vi "SwapInstanceVIUnusedName2 69.vi"(6 "Bindata & descr in":T1, 7 "type":cdb, 8 "error in (no error)":errorcluster, 9 "dims":u8=3 min=1 max=3, 11 "kwarg_name":string="testarg") -> (0 "error out":errorcluster, 1 "Array 3D":cdb[][][](array[numeric]) format="%.2f", 2 "Array 2D":cdb[][](array[numeric]) format="%.2f", 3 "Array 1D":cdb[](array[numeric]) format="%.2f", 4 "Bindata & descr out":T1, 5 "bindata":u8[](array[numeric]))   [LabVIEW 2018]
uses:
  Bindata&description.ctl
  Bindata description.ctl
  bdcbfef1-0b46-4e56-956b-efd7e52a8352.vi
  ec4bf352-c22a-4021-8efd-577ac70aacaa.vi
  66b8b619-fbe3-45a4-a1cc-203eb9b1f5dc.vi
  f262bfa0-5f14-49db-af0c-aad155b06c38.vi
  ec4bf352-c22a-4021-8efd-577ac70aacaa.vi/961f97e1-d54a-4e62-be37-74572e5b9f83.vi
  66b8b619-fbe3-45a4-a1cc-203eb9b1f5dc.vi/5bdaa807-7911-40a4-928e-6d0b25e11cf6.vi
  f262bfa0-5f14-49db-af0c-aad155b06c38.vi/a331fc70-2e34-4be0-817e-a64d7f4c7d79.vi
  ec4bf352-c22a-4021-8efd-577ac70aacaa.vi/961f97e1-d54a-4e62-be37-74572e5b9f83.vi/a85859f1-6a01-45ef-8e4c-231faaeaae98.vi
  66b8b619-fbe3-45a4-a1cc-203eb9b1f5dc.vi/5bdaa807-7911-40a4-928e-6d0b25e11cf6.vi/e5bad492-59a7-411a-a4a3-726d696f4125.vi
  f262bfa0-5f14-49db-af0c-aad155b06c38.vi/a331fc70-2e34-4be0-817e-a64d7f4c7d79.vi/75280eb0-2824-4b96-8a24-41904d7d4e2c.vi
  ec4bf352-c22a-4021-8efd-577ac70aacaa.vi/961f97e1-d54a-4e62-be37-74572e5b9f83.vi/a85859f1-6a01-45ef-8e4c-231faaeaae98.vi/9d1e86aa-c211-4185-9eac-3e06c0eb4835.vi
  66b8b619-fbe3-45a4-a1cc-203eb9b1f5dc.vi/5bdaa807-7911-40a4-928e-6d0b25e11cf6.vi/e5bad492-59a7-411a-a4a3-726d696f4125.vi/91efaebe-290b-41fc-a773-0eb7a6083b7d.vi
  f262bfa0-5f14-49db-af0c-aad155b06c38.vi/a331fc70-2e34-4be0-817e-a64d7f4c7d79.vi/75280eb0-2824-4b96-8a24-41904d7d4e2c.vi/24bfebee-2e4b-4f78-9251-0a951621d460.vi
  check ID validity.vi
  LV-Julia_ZMQ-Roundtrip_lib.lvlib
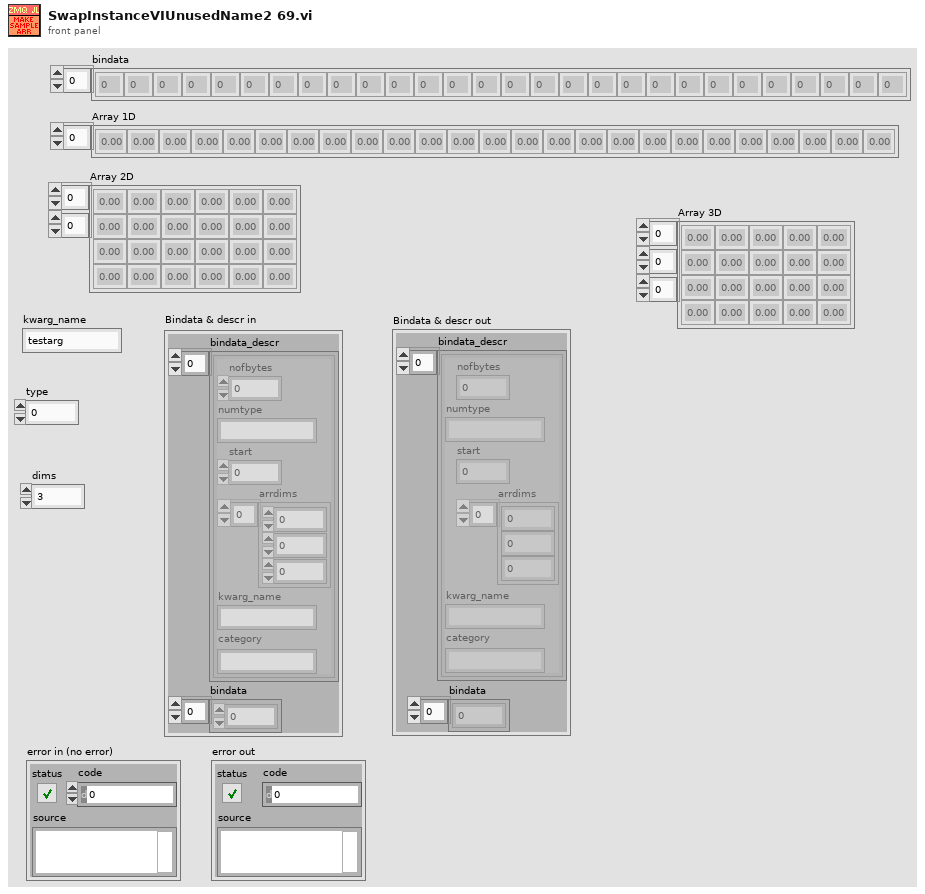
[diagram p1: front panel]
types:
  T1 = typedef "Bindata&description.ctl" = cluster{"bindata_descr":T2[], "bindata":u8[]}
  T2 = typedef "LV-Julia_ZMQ-Roundtrip_lib.lvlib/Bindata description.ctl" = cluster{"nofbytes":i32, "numtype":string, "start":i32, "arrdims":i32[], "kwarg_name":string, "category":string}
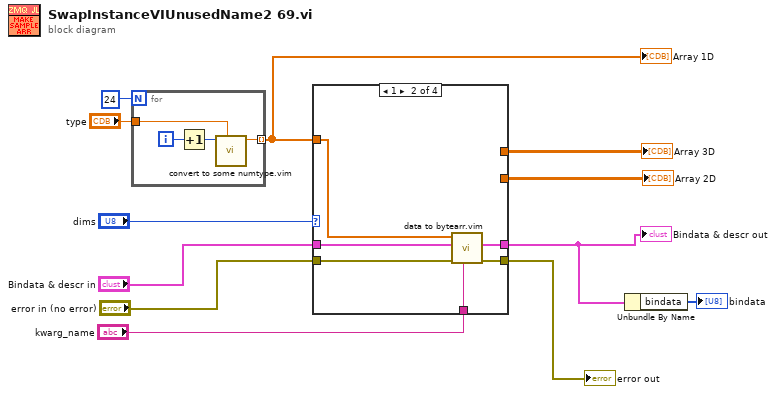
[diagram p0: block diagram]
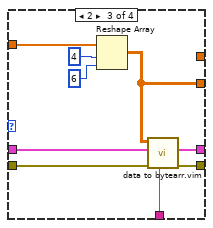
[diagram p3: hidden frame]
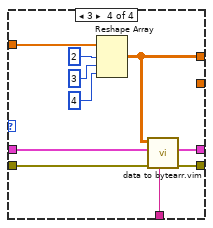
[diagram p4: hidden frame]
diagram:
  n1 = for {
    N: 24 -> [_]
    tunnel: [w14] -> w11 mode=indexing
    tunnel: "type" -> [w13]
    i -> [w16]
    n2 = Increment(x=w16) -> (x+1=w15:i32)
    n3 = call "convert to some numtype.vim"("type"=w13, "Numeric in"=w15) -> ("Numeric out"=w14:cdb)  [unwired: 9 in]
  }
  "Array 1D" <- w11
  n4 = case shown="1" "dims" {
    tunnel: [_ _ _ w42] -> w12
    tunnel: w11 -> [_ w23 w30 w38]
    tunnel: "kwarg_name" -> [_ w22 w29 w37]
    tunnel: "error in (no error)" -> [w17 w21 w28 w36]
    tunnel: [w17 w20 w27 w35] -> w5
    tunnel: [_ w19 w26 w34] -> w2
    tunnel: [_ _ w25 _] -> w4
    tunnel: "Bindata & descr in" -> [_ w18 w24 w33]
    frame 0, Default {
    }
    frame 1 {
      n5 = call "data to bytearr.vim"("kwarg_name"=w22, "error in (no error)"=w21, "Bindata & descr in"=w18, "data in"=w23) -> ("error out"=w20:errorcluster, "Bindata & descr out"=w19:T1)  [unwired: 5 in, 1 out]
    }
    frame 2 {
      n6 = Reshape Array(w30, 4 ("dimension size"), 6 ("dimension size")) -> (w25:cdb[][])
      n7 = call "data to bytearr.vim"("kwarg_name"=w29, "error in (no error)"=w28, "Bindata & descr in"=w24, "data in"=w25) -> ("error out"=w27:errorcluster, "Bindata & descr out"=w26:T1)  [unwired: 5 in, 1 out]
    }
    frame 3 {
      n8 = Reshape Array(w38, 2 ("dimension size"), 3 ("dimension size"), 4 ("dimension size")) -> (w42:cdb[][][])
      n9 = call "data to bytearr.vim"("kwarg_name"=w37, "error in (no error)"=w36, "Bindata & descr in"=w33, "data in"=w42) -> ("error out"=w35:errorcluster, "Bindata & descr out"=w34:T1)  [unwired: 5 in, 1 out]
    }
  }
  "Array 3D" <- w12
  "Bindata & descr out" <- w2
  "error out" <- w5
  "Array 2D" <- w4
  n10 = Unbundle By Name(w2) -> ("bindata"=→"bindata":u8[])
